vi "delete mapping by action channel.vi"(7 "owner ID":string, 8 "error in":errorcluster, 10 "action channel":refnum<class "TBM channel.lvclass">, 11 "engine configuration in":refnum<class "base TBM sequencer configuration.lvclass">) -> (0 "error out":errorcluster, 3 "engine configuration out":refnum<class "base TBM sequencer configuration.lvclass">)   [LabVIEW 2014, in "base TBM sequencer configuration.lvclass"]
uses:
  base TBM sequencer configuration.lvclass
  <vilib>/NI/Tag Bus Module Framework/channel/TBM channel.lvclass
  <vilib>/NI/Configuration Framework/NISE_CEF_TreeControl.lvlib
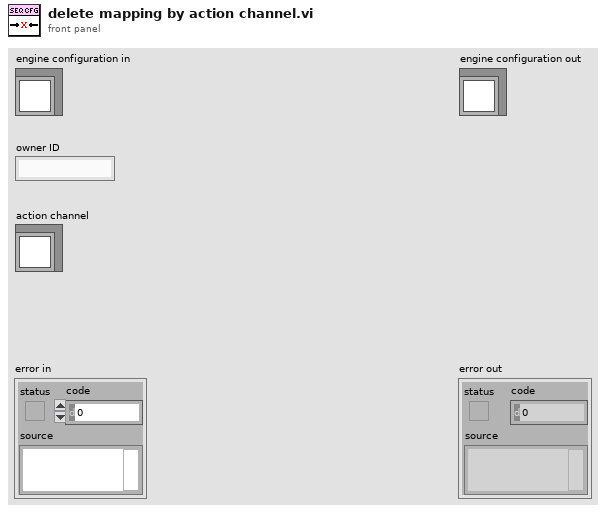
[diagram p1: front panel]
types:
  T1 = typedef "tag bus.lvlib/data table.lvlib/mapping specification.ctl" = cluster{"data type":T2, "mappings":T3[]}
  T2 = typedef "tag bus.lvlib/tag descriptor.lvclass/Data Type.ctl" = enum16{"Double", "Single", "I64", "I32", "I16", "I8", "U64", "U32", "U16", "U8", "Boolean", "String", "Array of Double", "Array of Single", "Array of I64", "Array of I32", "Array of I16", "Array of I8", "Array of U64", "Array of U32", "Array of U16", "Array of U8", "Array of Boolean", "Array of String"}
  T3 = typedef "tag bus.lvlib/data table.lvlib/mapping.ctl" = cluster{"sink name":string, "source name":string}
  T4 = typedef "TBM channel.lvclass/channel classification.ctl" = enum16{"input data", "output data", "processing parameter", "processing result"}
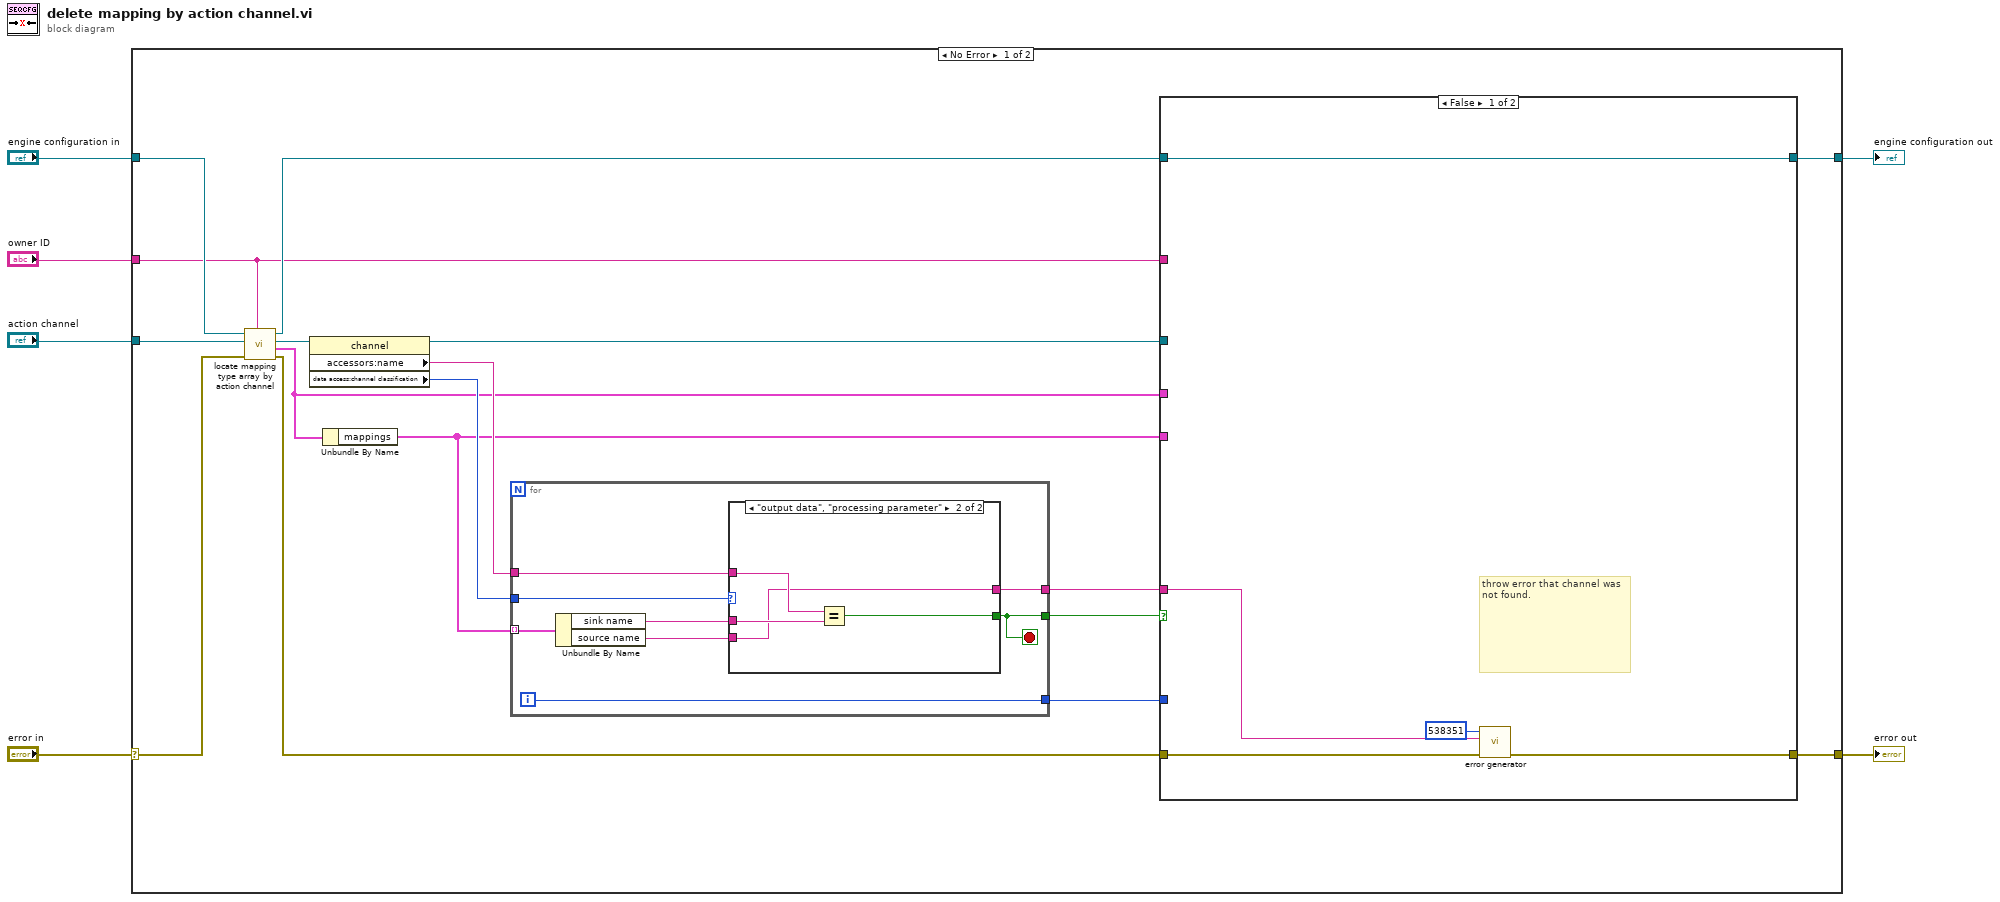
[diagram p0: block diagram]
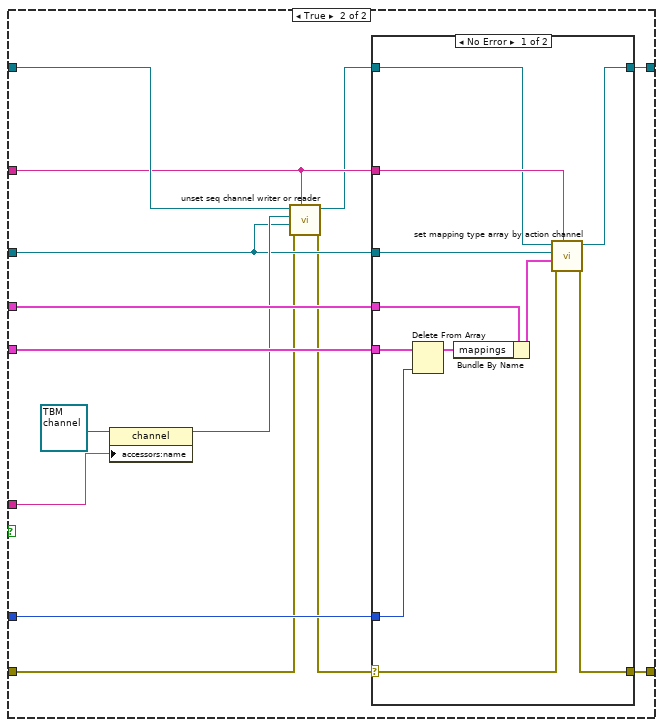
[diagram p2: hidden frame]
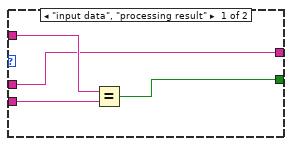
[diagram p4: hidden frame]
diagram:
  n1 = case shown="No Error" "error in" {
    selector: "error in" -> [w12 w73]
    tunnel: [w23 w73] -> w5
    tunnel: [w22 w72] -> w3
    tunnel: "engine configuration in" -> [w15 w72]
    tunnel: "owner ID" -> [w8 _]
    tunnel: "action channel" -> [w13 _]
    frame No Error {
      n2 = call "locate mapping type array by action channel.vi"("owner ID"=w8, "error in"=w12, "action channel"=w13, "engine configuration in"=w15) -> ("error out"=w11:errorcluster, "Mapping"=w9:T1, "action channel out"=w10:refnum<class "TBM channel.lvclass">, "engine configuration out"=w14:refnum<class "base TBM sequencer configuration.lvclass">)  [unwired: 4 in]
      n3 = property class="channel"(reference=w10) -> (reference out=w16:refnum<class "TBM channel.lvclass">, "accessors:name"=w20:string, "data access:channel classification"=w21:T4)  [unwired: 1 in, 1 out]
      n4 = Unbundle By Name(w9) -> ("mappings"=w17:T3[])
      n5 = for {
        tunnel: w17 -> [w63] mode=indexing
        tunnel: w21 -> [w62]
        tunnel: w20 -> [w59]
        tunnel: [w58] -> w19
        tunnel: [w57] -> w18
        tunnel: [w56] -> w7
        i -> [w57]
        stop <- w58 stop-if-true
        n6 = Unbundle By Name(w63) -> ("sink name"=w61:string, "source name"=w60:string)
        n7 = case shown="\"output data\", \"processing parameter\"" w62 {
          tunnel: w61 -> [w64 w70]
          tunnel: w60 -> [w67 w68]
          tunnel: w59 -> [w66 w71]
          tunnel: [w65 w69] -> w58
          tunnel: [w64 w68] -> w56
          frame "input data", "processing result" {
            n8 = Equal?(x=w66, y=w67) -> (x = y?=w65:bool)
          }
          frame "output data", "processing parameter" {
            n9 = Equal?(x=w71, y=w70) -> (x = y?=w69:bool)
          }
        }
      }
      n10 = case shown="False" w19 {
        tunnel: w11 -> [w26 w31]
        tunnel: w18 -> [_ w41]
        tunnel: w17 -> [_ w42]
        tunnel: w9 -> [_ w40]
        tunnel: w16 -> [_ w32]
        tunnel: w14 -> [w28 w35]
        tunnel: [w28 w39] -> w22
        tunnel: [w24 w38] -> w23
        tunnel: w8 -> [_ w34]
        tunnel: w7 -> [w25 w36]
        frame False {
          # "throw error that channel was not found."
          n11 = call <vilib>:"error generator.vi"("error in"=w26, "append error message"=w25, "error code (0)"=538351) -> ("error out"=w24:errorcluster)  [unwired: 6 in]
        }
        frame True {
          n12 = property class="channel"(reference=refnum<class "TBM channel.lvclass"> refnum ("tag descriptor"), "accessors:name"=w36) -> (reference out=w33:refnum<class "TBM channel.lvclass">)  [unwired: 1 in, 1 out]
          n13 = call "unset seq channel writer or reader.vi"("action GUID"=w34, "error in"=w31, "action channel"=w32, "seq channel"=w33, "engine configuration in"=w35) -> ("error out"=w30:errorcluster, "engine configuration out"=w29:refnum<class "base TBM sequencer configuration.lvclass">)  [unwired: 5 in]
          n14 = case shown="No Error" w30 {
            selector: w30 -> [w44 w54]
            tunnel: w42 -> [w53 _]
            tunnel: w41 -> [w52 _]
            tunnel: w40 -> [w51 _]
            tunnel: [w48 w55] -> w39
            tunnel: [w47 w54] -> w38
            tunnel: w34 -> [w46 _]
            tunnel: w32 -> [w45 _]
            tunnel: w29 -> [w43 w55]
            frame No Error {
              n15 = Delete From Array(array=w53, index=w52) -> (array with subset deleted=w50:T3[])  [unwired: 1 in, 1 out]
              n16 = Bundle By Name(cluster=w51, "mappings"=w50) -> (w49:T1)
              n17 = call "set mapping type array by action channel.vi"("owner ID"=w46, "error in"=w44, "Mapping"=w49, "action channel"=w45, "engine configuration in"=w43) -> ("error out"=w47:errorcluster, "engine configuration out"=w48:refnum<class "base TBM sequencer configuration.lvclass">)  [unwired: 5 in]
            }
            frame Error {
            }
          }
        }
      }
    }
    frame Error {
    }
  }
  "error out" <- w5
  "engine configuration out" <- w3
